vi "DAQmx Read (Counter Pulse Time 1Chan 1Samp).vi"(0 "task/channels in":refnum<k21>, 9 "timeout":dbl=10.0 format="%0.2f", 11 "error in":errorcluster) -> (4 "task out":refnum<k21>, 6 "high time":dbl, 8 "low time":dbl, 15 "error out":errorcluster)   [LabVIEW 2013]
doc: "Reads a single pair of pulse high and low times from a counter input task."
uses:
  nilvaiu.dll
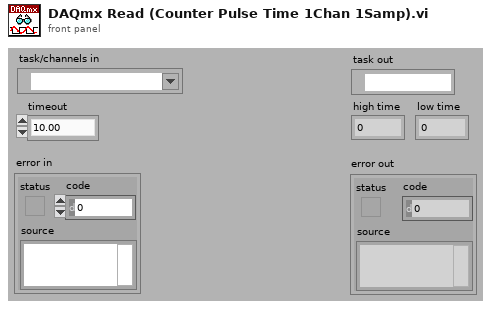
[diagram p1: front panel]
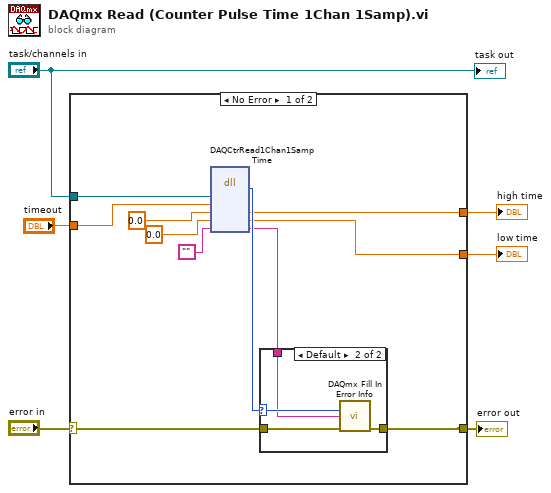
[diagram p0: block diagram]
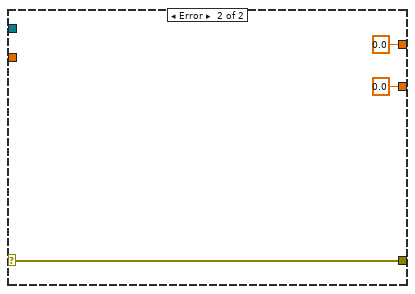
[diagram p3: hidden frame]
diagram:
  n1 = case shown="No Error" "error in" {
    selector: "error in" -> [w13 w25]
    tunnel: [w16 w25] -> w5
    tunnel: "task/channels in" -> [w17 _]
    tunnel: [w14 0.0 ("freq")] -> w3
    tunnel: "timeout" -> [w12 _]
    tunnel: [w7 0.0 ("freq")] -> w1
    frame No Error {
      n2 = dll-call lib="nilvaiu.*" fn="DAQCtrRead1Chan1SampTime"("taskID"=w17, "timeout"=w12, "highTime"=0.0 ("freq"), "lowTime"=0.0 ("freq"), "extendedErrorInfo"="") -> ("return type"=w15:i32, "highTime"=w14:dbl, "lowTime"=w7:dbl, "extendedErrorInfo"=w8:string)  [unwired: 4 in, 3 out]
      n3 = case shown="Default" w15 {
        selector: w15 -> [_ w20]
        tunnel: w13 -> [w18 w22]
        tunnel: [w18 w21] -> w16
        tunnel: w8 -> [_ w19]
        frame 0 {
        }
        frame Default {
          n4 = call "DAQmx Fill In Error Info.vi"("status code"=w20, "extended error info"=w19, "error in"=w22) -> ("error out"=w21:errorcluster)  [unwired: 1 in, 11 out]
        }
      }
    }
    frame Error {
    }
  }
  "error out" <- w5
  "high time" <- w3
  "low time" <- w1
  "task out" <- "task/channels in"
